vi "SIM BDF Eval Error.vi"(0 "outputs":dbl[](array[numeric]), 1 "min float":dbl, 2 "max step ratio":dbl, 5 "step size":dbl, 7 "proposed step size":dbl, 9 "min step size":dbl, 11 "BDF data":T1, 12 "max step size":dbl, 13 "relative tolerance":dbl, 14 "absolute tolerance":dbl) -> (3 "proposed new order out":i32, 4 "outputs out":dbl[](array[numeric]), 6 "step accepted? out":bool, 8 "proposed max step ratio out":dbl, 10 "proposed step size out":dbl, 15 "BDF data out":T1)   [LabVIEW 2018]
uses:
  SIM BDF data.ctl
  SIM Factored Matrix.ctl
  SIM BDF stages.ctl
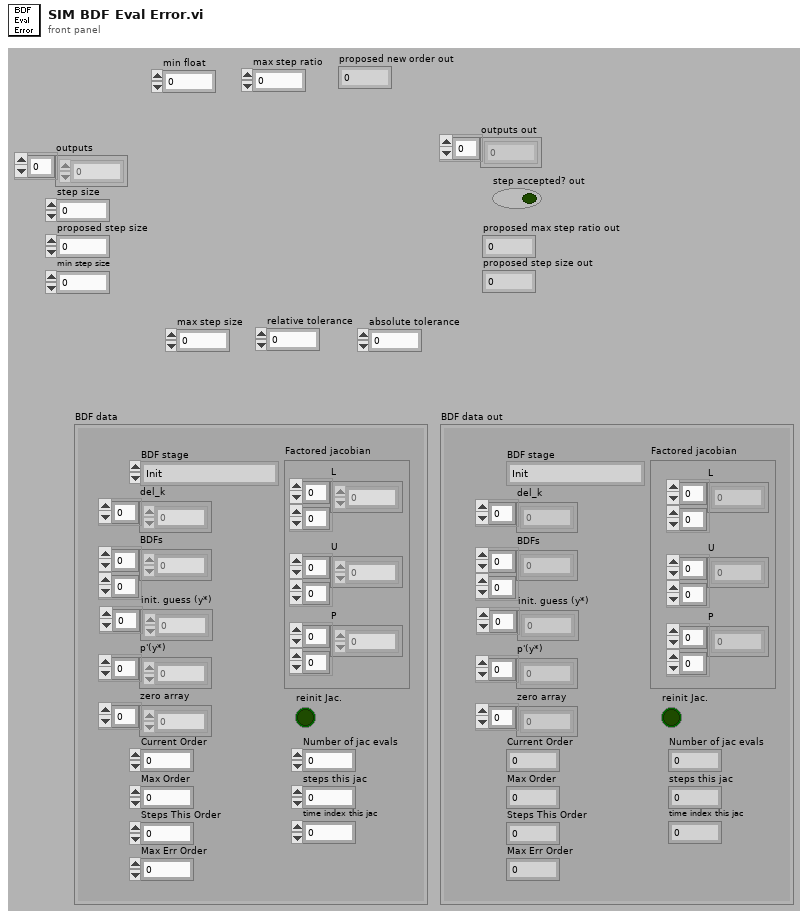
[diagram p1: front panel]
types:
  T1 = typedef "SIM BDF data.ctl" = cluster{"BDFs":dbl[][], "init. guess (y*)":dbl[], "p'(y*)":dbl[], "Factored jacobian":T2, "zero array":dbl[], "reinit Jac.":bool, "BDF stage":T3, "steps this jac":i32, "time index this jac":i32, "Number of jac evals":i32, "del_k":dbl[], "Current Order":i32, "Max Order":i32, "Steps This Order":i32, "Max Err Order":i32}
  T2 = typedef "SIM Factored Matrix.ctl" = cluster{"L":dbl[][], "U":dbl[][], "P":i32[][]}
  T3 = typedef "SIM BDF stages.ctl" = enum16{"Init", "Initial Guess", "Compute Jacobian", "Newton Iteration", "Eval Error", "Choose StepSize", "Reset BDFs"}
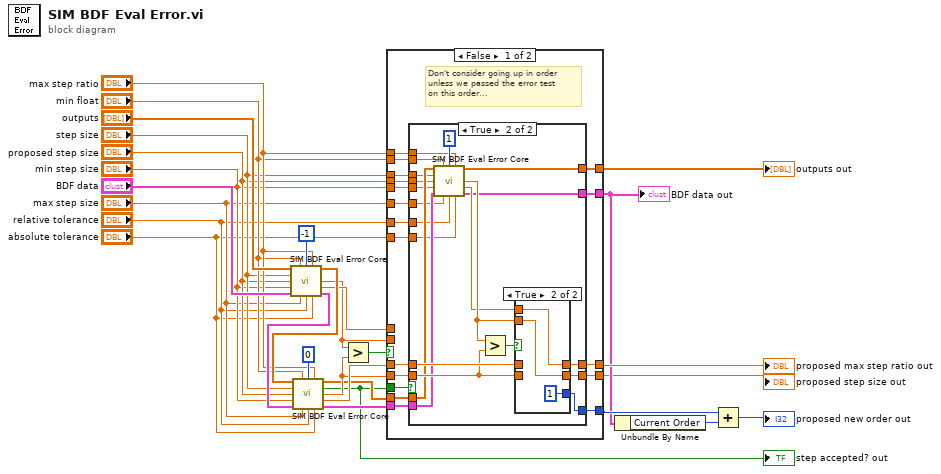
[diagram p0: block diagram]
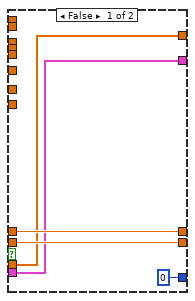
[diagram p2: hidden frame]
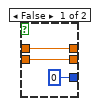
[diagram p3: hidden frame]
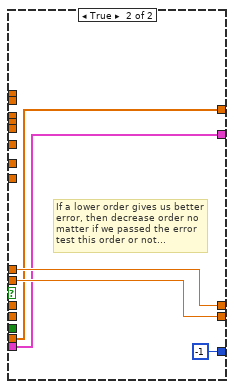
[diagram p4: hidden frame]
diagram:
  n1 = call "SIM BDF Eval Error Core.vi"("outputs"="outputs", "min float"="min float", "Delta Method Order"=-1, "max step ratio"="max step ratio", "step size"="step size", "proposed step size"="proposed step size", "min step size"="min step size", "BDF data"="BDF data", "max step size"="max step size", "relative tolerance"="relative tolerance", "absolute tolerance"="absolute tolerance") -> ("outputs out"=w26:dbl[], "proposed step size out"=w18:dbl, "proposed max step ratio"=w19:dbl, "BDF data out"=w25:T1)  [unwired: 1 out]
  n2 = call "SIM BDF Eval Error Core.vi"("outputs"=w26, "min float"="min float", "Delta Method Order"=0, "max step ratio"="max step ratio", "step size"="step size", "proposed step size"="proposed step size", "min step size"="min step size", "BDF data"=w25, "max step size"="max step size", "relative tolerance"="relative tolerance", "absolute tolerance"="absolute tolerance") -> ("outputs out"=w13:dbl[], "step accepted? out"=w4:bool, "proposed step size out"=w16:dbl, "proposed max step ratio"=w17:dbl, "BDF data out"=w12:T1)
  "step accepted? out" <- w4
  n3 = Greater?(x=w18, y=w16) -> (0:w23:bool)
  n4 = case shown="False" w23 {
    tunnel: w19 -> [_ w84]
    tunnel: w17 -> [w45 _]
    tunnel: w16 -> [w47 _]
    tunnel: w18 -> [_ w83]
    tunnel: w4 -> [w46 _]
    tunnel: [w44 -1] -> w21
    tunnel: [w43 w84] -> w22
    tunnel: [w42 w83] -> w1
    tunnel: "max step ratio" -> [w41 _]
    tunnel: "min float" -> [w40 _]
    tunnel: w13 -> [w39 w81]
    tunnel: w12 -> [w38 w80]
    tunnel: "step size" -> [w37 _]
    tunnel: "proposed step size" -> [w36 _]
    tunnel: "min step size" -> [w35 _]
    tunnel: "max step size" -> [w34 _]
    tunnel: "relative tolerance" -> [w33 _]
    tunnel: "absolute tolerance" -> [w32 _]
    tunnel: [w31 w80] -> w3
    tunnel: [w30 w81] -> w5
    frame False {
      # "Don't consider going up in order\nunless we passed the error test\non this order..."
      n5 = case shown="True" w46 {
        tunnel: w47 -> [w50 w71]
        tunnel: w45 -> [w51 w72]
        tunnel: [0 w70] -> w44
        tunnel: [w51 w69] -> w43
        tunnel: [w50 w68] -> w42
        tunnel: w41 -> [_ w66]
        tunnel: w40 -> [_ w65]
        tunnel: w39 -> [w49 w64]
        tunnel: w38 -> [w48 w63]
        tunnel: w37 -> [_ w62]
        tunnel: w36 -> [_ w61]
        tunnel: w35 -> [_ w60]
        tunnel: w34 -> [_ w59]
        tunnel: w33 -> [_ w58]
        tunnel: w32 -> [_ w57]
        tunnel: [w48 w54] -> w31
        tunnel: [w49 w53] -> w30
        frame False {
        }
        frame True {
          n6 = call "SIM BDF Eval Error Core.vi"("outputs"=w64, "min float"=w65, "Delta Method Order"=1, "max step ratio"=w66, "step size"=w62, "proposed step size"=w61, "min step size"=w60, "BDF data"=w63, "max step size"=w59, "relative tolerance"=w58, "absolute tolerance"=w57) -> ("outputs out"=w53:dbl[], "proposed step size out"=w56:dbl, "proposed max step ratio"=w55:dbl, "BDF data out"=w54:T1)  [unwired: 1 out]
          n7 = Greater?(x=w56, y=w71) -> (0:w73:bool)
          n8 = case shown="True" w73 {
            tunnel: w56 -> [_ w78]
            tunnel: w55 -> [_ w79]
            tunnel: w72 -> [w76 _]
            tunnel: w71 -> [w75 _]
            tunnel: [w76 w79] -> w69
            tunnel: [w75 w78] -> w68
            tunnel: [0 1] -> w70
            frame False {
            }
            frame True {
            }
          }
        }
      }
    }
    frame True {
      # "If a lower order gives us better\nerror, then decrease order no\nmatter if we passed the error \ntest this order or not..."
    }
  }
  "proposed max step ratio out" <- w22
  "proposed step size out" <- w1
  "outputs out" <- w5
  "BDF data out" <- w3
  n9 = Unbundle By Name(w3) -> ("Current Order"=w2:i32)
  n10 = Add(x=w21, y=w2) -> (x+y=→"proposed new order out":i32)
